vi "Initialize Transfer Groups.vi"(8 "error in (no error)":errorcluster, 10 "Transfer Group Configurations":T1[](array[typedef]) {"Transfers"."channels"."string offset" format="%d bytes"}, 11 "UDP Transceiver in":refnum<class "UDP Transceiver.lvclass">) -> (0 "error out":errorcluster, 3 "UDP Transceiver out":refnum<class "UDP Transceiver.lvclass">)   [LabVIEW 2017, in "UDP.lvlib" / "UDP Transceiver.lvclass"]
uses:
  UDP Transceiver.lvclass
  Builds/Data Sharing Framework/Current/Core/DSF Core.lvlibp/Typedefs/DSF Engine Transfer Group Configuration.ctl
  Builds/Data Sharing Framework/Current/Core/DSF Core.lvlibp/Typedefs/DSF Direction.ctl
  Builds/Data Sharing Framework/Current/Core/DSF Core.lvlibp/Typedefs/DSF Timing Info.ctl
  Builds/Data Sharing Framework/Current/Core/DSF Core.lvlibp/Typedefs/DSF Settings Info.ctl
  Builds/Data Sharing Framework/Current/Core/DSF Core.lvlibp/Typedefs/DSF Engine Transfer Configuration.ctl
  Builds/Data Sharing Framework/Current/Core/DSF Core.lvlibp/Typedefs/DSF Byte Order.ctl
  Builds/Data Sharing Framework/Current/Core/DSF Core.lvlibp/Typedefs/DSF Engine Channel Configuration.ctl
  Builds/Data Sharing Framework/Current/Core/DSF Core.lvlibp/Typedefs/DSF Data Type.ctl
  Builds/Data Sharing Framework/Current/Core/DSF Core.lvlibp/Typedefs/DSF Timeout Behavior.ctl
  UDP Transceiver.lvclass/UDP Transceiver.ctl
  Transfer Group Parameters.ctl
  Transfer Group Rx Parameters.ctl
  Transfer Rx Parameters.ctl
  Transfer Group Tx Parameters.ctl
  Transfer Tx Parameters.ctl
  Builds/Data Sharing Framework/Current/Core/DSF Core.lvlibp/Classes/Configuration/Required Buffer Size (Transfer).vi
  Builds/Data Sharing Framework/Current/Core/DSF Core.lvlibp/Classes/Configuration/Configuration Session.lvclass
  Builds/Data Sharing Framework/Current/Core/DSF Core.lvlibp
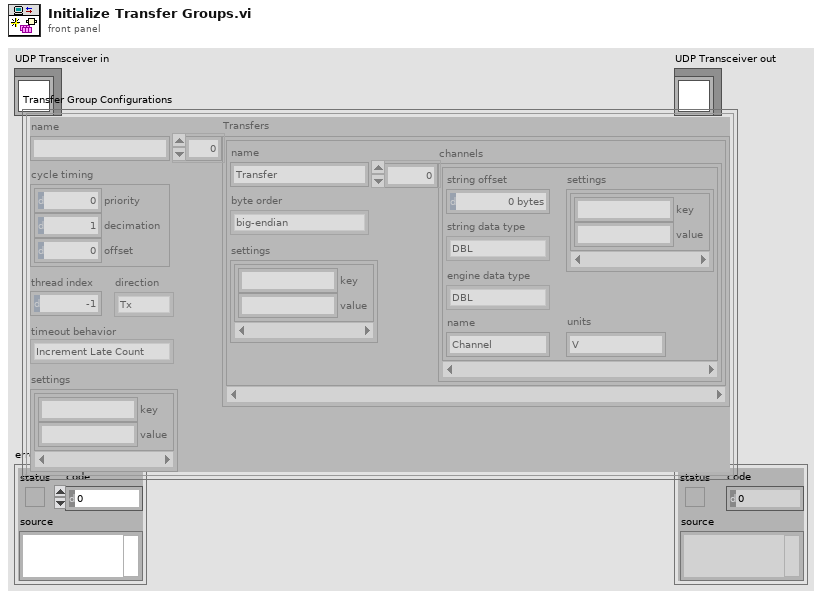
[diagram p1: front panel]
types:
  T1 = typedef "DSF Core.lvlibp/DSF Engine Transfer Group Configuration.ctl" = cluster{"name":string, "direction":T2, "cycle timing":T3, "thread index":i32, "settings":T4, "Transfers":T5[], "timeout behavior":T9}
  T2 = typedef "DSF Core.lvlibp/DSF Direction.ctl" = enum8{"Tx", "Rx"}
  T3 = typedef "DSF Core.lvlibp/DSF Timing Info.ctl" = cluster{"priority":u64, "decimation":u64, "offset":u64}
  T4 = typedef "DSF Core.lvlibp/DSF Settings Info.ctl" = cluster{"key":string, "value":string}[]
  T5 = typedef "DSF Core.lvlibp/DSF Engine Transfer Configuration.ctl" = cluster{"name":string, "byte order":T6, "settings":T4, "channels":T7[]}
  T6 = typedef "DSF Core.lvlibp/DSF Byte Order.ctl" = enum8{"big-endian", "little-endian"}
  T7 = typedef "DSF Core.lvlibp/DSF Engine Channel Configuration.ctl" = cluster{"string offset":u64, "string data type":T8, "engine data type":T8, "name":string, "settings":T4, "units":string}
  T8 = typedef "DSF Core.lvlibp/DSF Data Type.ctl" = enum8{"Bool", "SGL", "DBL", "I8", "I16", "I32", "I64", "U8", "U16", "U32", "U64"}
  T9 = typedef "DSF Core.lvlibp/DSF Timeout Behavior.ctl" = enum8{"Increment Late Count", "Throw Error"}
  T10 = typedef "UDP.lvlib/UDP Transceiver.lvclass/Transfer Group Parameters.ctl" = cluster{"Rx":T11, "Tx":T13}
  T11 = typedef "UDP.lvlib/UDP Transceiver.lvclass/Transfer Group Rx Parameters.ctl" = cluster{"Transfers Rx":T12[], "max size":i32}
  T12 = typedef "UDP.lvlib/UDP Transceiver.lvclass/Transfer Rx Parameters.ctl" = cluster{"timeout":i32, "source address":u32, "source port":u16}
  T13 = typedef "UDP.lvlib/UDP Transceiver.lvclass/Transfer Group Tx Parameters.ctl" = cluster{"Transfers Tx":T14[]}
  T14 = typedef "UDP.lvlib/UDP Transceiver.lvclass/Transfer Tx Parameters.ctl" = cluster{"destination port":u16, "destination address":u32}
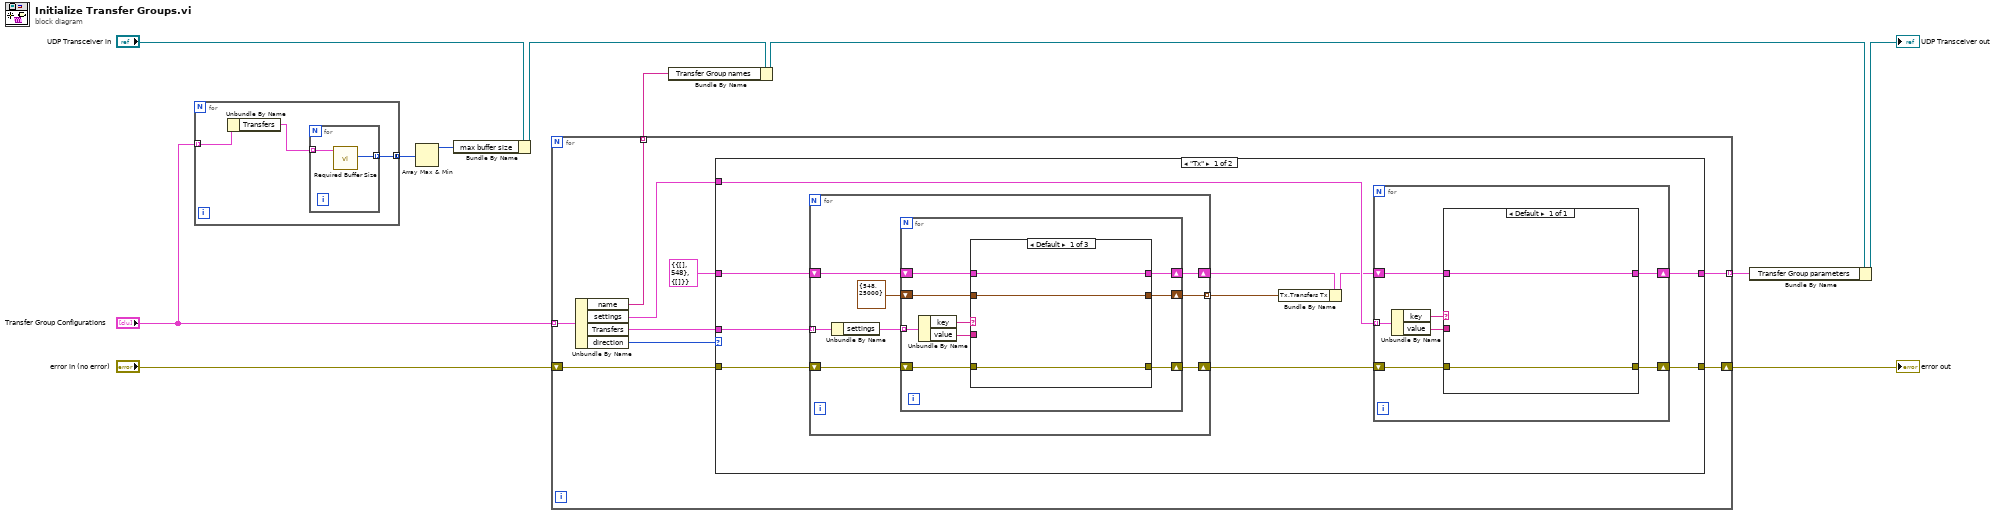
[diagram p0: block diagram]
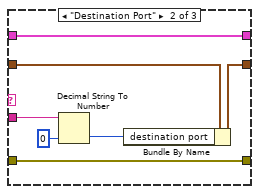
[diagram p2: hidden frame]
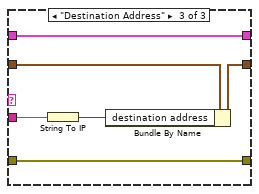
[diagram p3: hidden frame]
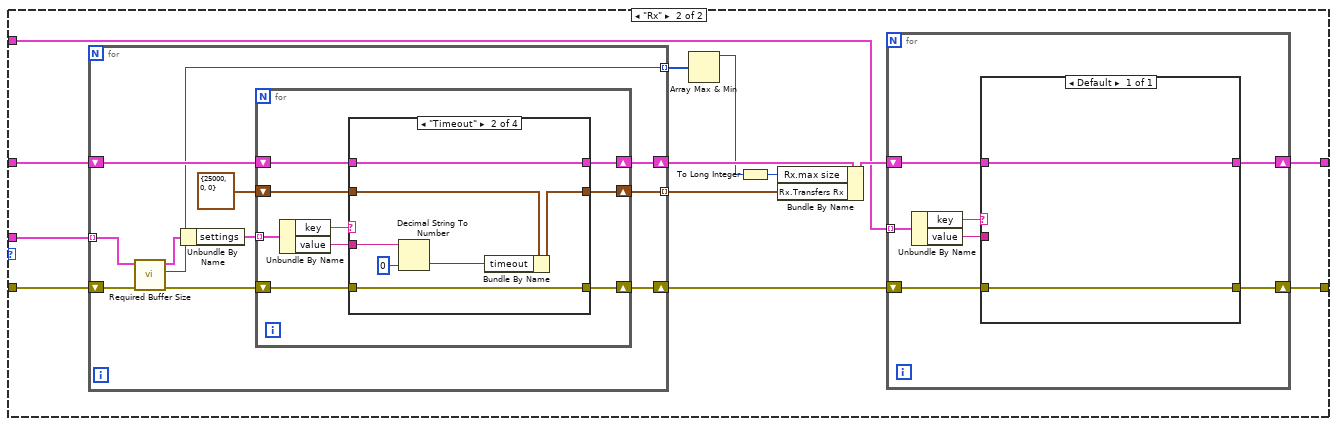
[diagram p4: hidden frame]
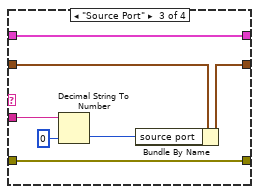
[diagram p6: hidden frame]
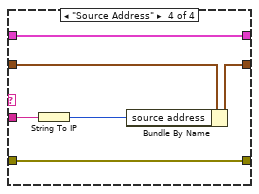
[diagram p7: hidden frame]
diagram:
  n1 = for {
    tunnel: "Transfer Group Configurations" -> [w13] mode=indexing
    tunnel: [w14] -> w11 mode=concatenating
    n2 = Unbundle By Name(w13) -> ("Transfers"=w12:T5[])
    n3 = for {
      tunnel: w12 -> [w16] mode=indexing
      tunnel: [w15] -> w14 mode=indexing
      n4 = call-poly "Required Buffer Size.vi"("Transfer Configuration in"=w16) -> ("string buffer size"=w15:u64)  [unwired: 7 in, 3 out]
    }
  }
  n5 = Array Max & Min(array=w11) -> (max value=w10:u64)  [unwired: 3 out]
  n6 = Bundle By Name(cluster="UDP Transceiver in", "max buffer size"=w10) -> (w9:refnum<class "UDP Transceiver.lvclass">)
  n7 = for {
    tunnel: "Transfer Group Configurations" -> [w21] mode=indexing
    tunnel: [w18] -> w8 mode=indexing
    tunnel: [w25] -> w6 mode=indexing
    shift-right: [w23] -> w1
    shift-left: "error in (no error)" -> [w24]
    n8 = Unbundle By Name(w21) -> ("name"=w18:string, "settings"=w17:T4, "Transfers"=w19:T5[], "direction"=w20:T2)
    n9 = case shown="\"Tx\"" w20 {
      tunnel: T10 {"Rx"={"Transfers Rx"=[], "max size"=548}, "Tx"={"Transfers Tx"=[]}} ("Rx/Tx Parameters") -> [w31 w85]
      tunnel: [w35 w90] -> w25
      tunnel: w24 -> [w33 w86]
      tunnel: [w34 w89] -> w23
      tunnel: w19 -> [w28 w79]
      tunnel: w17 -> [w27 w78]
      frame "Tx" {
        n10 = for {
          shift-right: [w42] -> w30
          shift-left: w31 -> [w43]
          shift-right: [w40] -> w32
          shift-left: w33 -> [w41]
          tunnel: w28 -> [w36] mode=indexing
          tunnel: [w38] -> w29 mode=indexing
          n11 = Unbundle By Name(w36) -> ("settings"=w37:T4)
          n12 = for {
            tunnel: w37 -> [w46] mode=indexing
            shift-right: [w49] -> w42
            shift-left: w43 -> [w50]
            shift-right: [w47] -> w40
            shift-left: w41 -> [w48]
            shift-right: [w45] -> w38
            shift-left: T14 {"destination port"=548, "destination address"=25000} ("Transfer Tx") -> [w44]
            n13 = Unbundle By Name(w46) -> ("key"=w52:string, "value"=w51:string)
            n14 = case shown="Default" w52 {
              tunnel: w51 -> [_ w62 w67]
              tunnel: w50 -> [w55 w57 w64]
              tunnel: [w55 w57 w64] -> w49
              tunnel: w48 -> [w54 w59 w68]
              tunnel: [w54 w59 w68] -> w47
              tunnel: w44 -> [w53 w58 w65]
              tunnel: [w53 w56 w63] -> w45
              frame Default {
              }
              frame "Destination Port" {
                n15 = Decimal String To Number(string=w62, default (0L)=u16 0 ("default (0 I32)")) -> (number=w60:u16)  [unwired: 1 in, 1 out]
                n16 = Bundle By Name(cluster=w58, "destination port"=w60) -> (w56:T14)
              }
              frame "Destination Address" {
                n17 = String To IP(1:w67) -> (0:w66:u32)
                n18 = Bundle By Name(cluster=w65, "destination address"=w66) -> (w63:T14)
              }
            }
          }
        }
        n19 = Bundle By Name(cluster=w30, "Tx.Transfers Tx"=w29) -> (w26:T10)
        n20 = for {
          tunnel: w27 -> [w73] mode=indexing
          shift-right: [w71] -> w35
          shift-left: w26 -> [w72]
          shift-right: [w69] -> w34
          shift-left: w32 -> [w70]
          n21 = Unbundle By Name(w73) -> ("key"=w75:string, "value"=w74:string)
          n22 = case shown="Default" w75 {
            tunnel: w74 -> [_]
            tunnel: w72 -> [w77]
            tunnel: [w77] -> w71
            tunnel: w70 -> [w76]
            tunnel: [w76] -> w69
            frame Default {
            }
          }
        }
      }
      frame "Rx" {
        n23 = for {
          shift-right: [w100] -> w88
          shift-left: w85 -> [w101]
          shift-right: [w99] -> w83
          shift-left: w86 -> [w93]
          tunnel: w79 -> [w95] mode=indexing
          tunnel: [w97] -> w87 mode=indexing
          tunnel: [w94] -> w82 mode=indexing
          n24 = call-poly "Required Buffer Size.vi"("error in (no error)"=w93, "Transfer Configuration in"=w95) -> ("error out"=w92:errorcluster, "string buffer size"=w94:u64, "Transfer Configuration out"=w91:T5)  [unwired: 6 in, 1 out]
          n25 = Unbundle By Name(w91) -> ("settings"=w96:T4)
          n26 = for {
            tunnel: w96 -> [w104] mode=indexing
            shift-right: [w107] -> w100
            shift-left: w101 -> [w108]
            shift-right: [w105] -> w99
            shift-left: w92 -> [w106]
            shift-right: [w103] -> w97
            shift-left: T12 {"timeout"=25000, "source address"=0, "source port"=0} ("Transfer Rx") -> [w102]
            n27 = Unbundle By Name(w104) -> ("key"=w110:string, "value"=w109:string)
            n28 = case shown="\"Timeout\"" w110 {
              tunnel: w109 -> [_ w120 w127 w129]
              tunnel: w108 -> [w113 w115 w122 w131]
              tunnel: [w113 w115 w122 w131] -> w107
              tunnel: w106 -> [w112 w117 w124 w133]
              tunnel: [w112 w117 w124 w133] -> w105
              tunnel: w102 -> [w111 w116 w123 w132]
              tunnel: [w111 w114 w121 w130] -> w103
              frame Default {
              }
              frame "Timeout" {
                n29 = Decimal String To Number(string=w120, default (0L)=0 ("default (0 I32)")) -> (number=w118:i32)  [unwired: 1 in, 1 out]
                n30 = Bundle By Name(cluster=w116, "timeout"=w118) -> (w114:T12)
              }
              frame "Source Port" {
                n31 = Decimal String To Number(string=w127, default (0L)=u16 0 ("default (0 I32)")) -> (number=w125:u16)  [unwired: 1 in, 1 out]
                n32 = Bundle By Name(cluster=w123, "source port"=w125) -> (w121:T12)
              }
              frame "Source Address" {
                n33 = String To IP(1:w129) -> (0:w128:u32)
                n34 = Bundle By Name(cluster=w132, "source address"=w128) -> (w130:T12)
              }
            }
          }
        }
        n35 = Array Max & Min(array=w82) -> (max value=w81:u64)  [unwired: 3 out]
        n36 = To Long Integer(number=w81) -> (32bit integer=w80:i32)
        n37 = Bundle By Name(cluster=w88, "Rx.max size"=w80, "Rx.Transfers Rx"=w87) -> (w84:T10)
        n38 = for {
          tunnel: w78 -> [w138] mode=indexing
          shift-right: [w136] -> w90
          shift-left: w84 -> [w137]
          shift-right: [w134] -> w89
          shift-left: w83 -> [w135]
          n39 = Unbundle By Name(w138) -> ("key"=w140:string, "value"=w139:string)
          n40 = case shown="Default" w140 {
            tunnel: w139 -> [_]
            tunnel: w137 -> [w142]
            tunnel: [w142] -> w136
            tunnel: w135 -> [w141]
            tunnel: [w141] -> w134
            frame Default {
            }
          }
        }
      }
    }
  }
  "error out" <- w1
  n41 = Bundle By Name(cluster=w9, "Transfer Group names"=w8) -> (w7:refnum<class "UDP Transceiver.lvclass">)
  n42 = Bundle By Name(cluster=w7, "Transfer Group parameters"=w6) -> (→"UDP Transceiver out":refnum<class "UDP Transceiver.lvclass">)
